vi "AutoEnumToString.vi"(10 "AutoEnum":i32) -> (2 "EnumString":string)   [LabVIEW 2012]
panel:
  in  "Array":string[](array[string])=["Disabled", "BackRight", "BackLeft", "CloseRight", "CloseLeft", "BehindPyramid"]
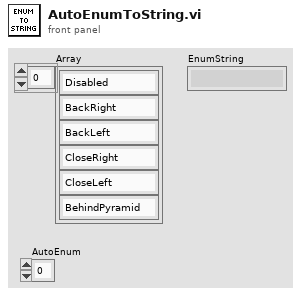
[diagram p1: front panel]
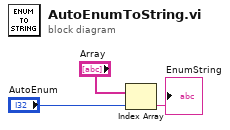
[diagram p0: block diagram]
diagram:
  n1 = Index Array(array="Array", index="AutoEnum") -> (element=→"EnumString":string)
